vi "Spark MAX_Get ALL Cached Parameter.vi"(8 "error in (no error)":errorcluster, 10 "Parameter ID":T2, 11 "SPARK MAX Device Ref in":T4) -> (0 "error out":errorcluster, 1 "Parameter Type":T3, 2 "Parameter Raw":u32, 3 "output cluster":T1 {"Float" format="%#_4f"}, 5 "Timestamp":u32)   [LabVIEW 2020]
uses:
  <vilib>/Rock Robotics/WPI/ThirdParty/REV Robotics/REVLib/Typedef/Spark MAX Parameter Type.ctl
  <vilib>/Rock Robotics/WPI/ThirdParty/REV Robotics/REVLib/Typedef/Spark MAX Parameter ID.ctl
  <vilib>/Rock Robotics/WPI/ThirdParty/REV Robotics/REVLib/Typedef/Spark MAX Variant Data.ctl
  Cluster_Spark Max parameter data.ctl
  <vilib>/Rock Robotics/WPI/ThirdParty/REV Robotics/REVLib/Typedef/Spark MAX Parameter Cache Element.ctl
  <vilib>/Rock Robotics/WPI/ThirdParty/REV Robotics/REVLib/Typedef/Spark MAX Parameter Status.ctl
panel:
  out "found":bool
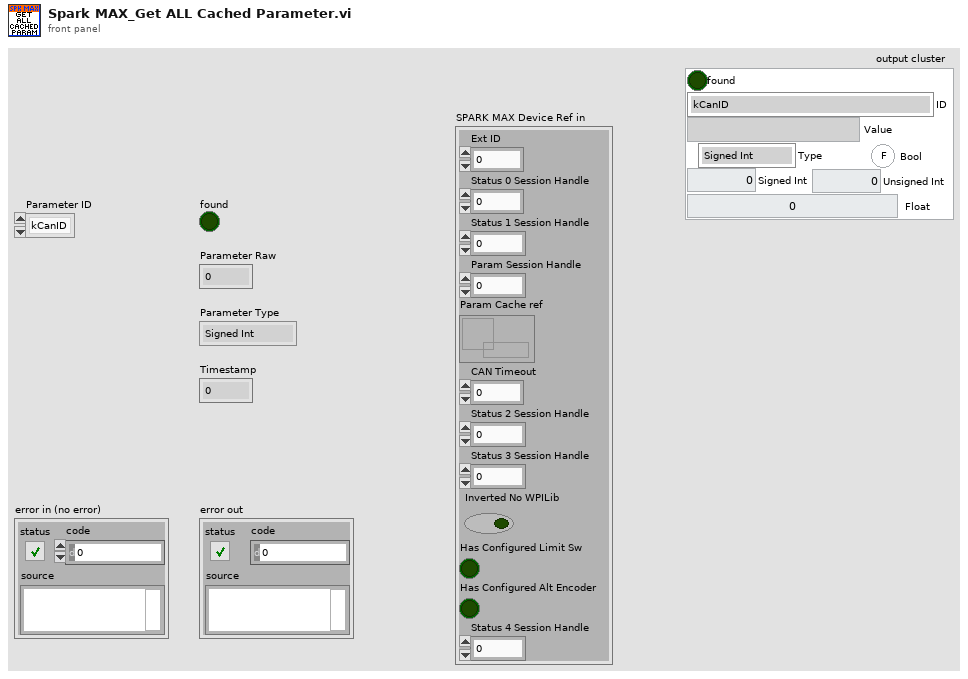
[diagram p1: front panel]
types:
  T1 = typedef "Cluster_Spark Max parameter data.ctl" = cluster{"found":bool, "ID":T2, "Value":string, "Type":T3, "Signed Int":i32, "Unsigned Int":u32, "Float":dbl, "Bool":bool}
  T2 = typedef "Spark MAX Parameter ID.ctl" = enum16{"kCanID", "kInputMode", "kMotorType", "kCommAdvance", "kSensorType", "kCtrlType", "kIdleMode", "kInputDeadband", "kFeedbackSensorPID0", "kFeedbackSensorPID1", "kPolePairs", "kCurrentChop", "kCurrentChopCycles", "kP_0", "kI_0", "kD_0", "kF_0", "kIZone_0", "kDFilter_0", "kOutputMin_0", "kOutputMax_0", "kP_1", "kI_1", "kD_1", "kF_1", "kIZone_1", "kDFilter_1", "kOutputMin_1", "kOutputMax_1", "kP_2", "kI_2", "kD_2", "kF_2", "kIZone_2", "kDFilter_2", "kOutputMin_2", "kOutputMax_2", "kP_3", "kI_3", "kD_3", "kF_3", "kIZone_3", "kDFilter_3", "kOutputMin_3", "kOutputMax_3", "kInverted", "kOutputRatio", "kSerialNumberLow", "kSerialNumberMid", "kSerialNumberHigh", "kLimitSwitchFwdPolarity", "kLimitSwitchRevPolarity", "kHardLimitFwdEn", "kHardLimitRevEn", "kSoftLimitFwdEn", "kSoftLimitRevEn", "kRampRate", "kFollowerID", "kFollowerConfig", "kSmartCurrentStallLimit", "kSmartCurrentFreeLimit", "kSmartCurrentConfig", "kSmartCurrentReserved", "kMotorKv", "kMotorR", "kMotorL", "kMotorRsvd1", "kMotorRsvd2", "kMotorRsvd3", "kEncoderCountsPerRev", "kEncoderAverageDepth", "kEncoderSampleDelta", "kEncoderInverted", "kEncoderRsvd1", "kClosedLoopVoltageMode", "kCompensatedNominalVoltage", "kSmartMotionMaxVelocity_0", "kSmartMotionMaxAccel_0", "kSmartMotionMinVelOutput_0", "kSmartMotionAllowedClosedLoopError_0", "kSmartMotionAccelStrategy_0", "kSmartMotionMaxVelocity_1", "kSmartMotionMaxAccel_1", "kSmartMotionMinVelOutput_1", "kSmartMotionAllowedClosedLoopError_1", "kSmartMotionAccelStrategy_1", "kSmartMotionMaxVelocity_2", "kSmartMotionMaxAccel_2", "kSmartMotionMinVelOutput_2", "kSmartMotionAllowedClosedLoopError_2", "kSmartMotionAccelStrategy_2", "kSmartMotionMaxVelocity_3", "kSmartMotionMaxAccel_3", "kSmartMotionMinVelOutput_3", "kSmartMotionAllowedClosedLoopError_3", "kSmartMotionAccelStrategy_3", "kIMaxAccum_0", "kSlot3Placeholder1_0", "kSlot3Placeholder2_0", "kSlot3Placeholder3_0", "kIMaxAccum_1", "kSlot3Placeholder1_1", "kSlot3Placeholder2_1", "kSlot3Placeholder3_1", "kIMaxAccum_2", "kSlot3Placeholder1_2", "kSlot3Placeholder2_2", "kSlot3Placeholder3_2", "kIMaxAccum_3", "kSlot3Placeholder1_3", "kSlot3Placeholder2_3", "kSlot3Placeholder3_3", "kPositionConversionFactor", "kVelocityConversionFactor", "kClosedLoopRampRate", "kSoftLimitFwd", "kSoftLimitRev", "kSoftLimitRsvd0", "kSoftLimitRsvd1", "kAnalogPositionConversion", "kAnalogVelocityConversion", "kAnalogAverageDepth", "kAnalogSensorMode", "kAnalogInverted", "kAnalogSampleDelta", "kAnalogRsvd0", "kAnalogRsvd1", "kDataPortConfig", "kAltEncoderCountsPerRev", "kAltEncoderAverageDepth", "kAltEncoderSampleDelta", "kAltEncoderInverted", "kAltEncoderPositionConversion", "kAltEncoderVelocityConversion", "kAltEncoderRsvd0", "kAltEncoderRsvd1", "kHallSensorSampleRate", "kHallSensorAverageDepth", "kNumParameters", "kDutyCyclePositionFactor", "kDutyCycleVelocityFactor", "kDutyCycleInverted", "kDutyCycleSensorMode", "kDutyCycleAverageDepth", "kDutyCycleSampleDelta", "kDutyCycleOffsetv1p6p2", "kDutyCycleRsvd0", "kDutyCycleRsvd1", "kDutyCycleRsvd2", "kPositionPIDWrapEnable", "kPositionPIDMinInput", "kPositionPIDMaxInput", "kDutyCycleZeroCentered", "kDutyCyclePrescalar", "kDutyCycleOffset"}
  T3 = typedef "Spark MAX Parameter Type.ctl" = enum16{"Signed Int", "Unsigned Int", "Float", "Bool"}
  T4 = typedef "Spark MAX Variant Data.ctl" = cluster{"Ext ID":u32, "Status 0 Session Handle":u32, "Status 1 Session Handle":u32, "Param Session Handle":u32, "Param Cache ref":refnum<data-value>, "CAN Timeout":u32, "Status 2 Session Handle":u32, "Status 3 Session Handle":u32, "Inverted No WPILib":bool, "Has Configured Limit Sw":bool, "Has Configured Alt Encoder":bool, "Status 4 Session Handle":u32}
  T5 = typedef "Spark MAX Parameter Status.ctl" = enum16{"Ok", "Invalid Parameter ID", "Mismatch Type", "Access Mode", "Invalid Parameter Value", "Not Implemented/Depcrecated"}
  T6 = typedef "Spark MAX Parameter Cache Element.ctl" = cluster{"Timestamp":u32, "Parameter Raw":u32, "Parameter Type":T3, "Last Access Status":T5}
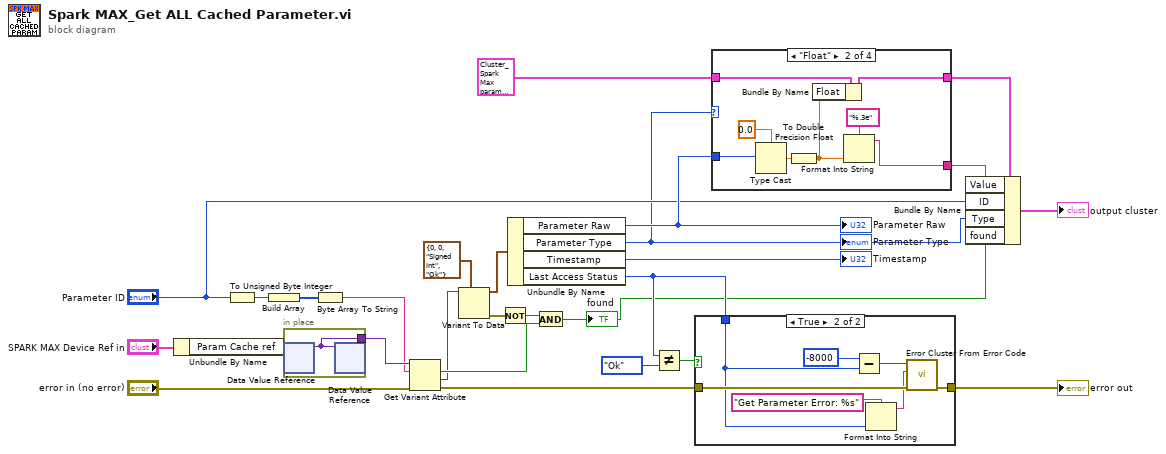
[diagram p0: block diagram]
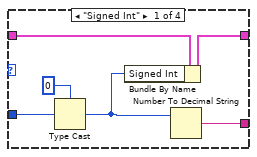
[diagram p2: hidden frame]
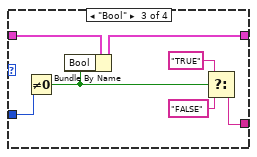
[diagram p3: hidden frame]
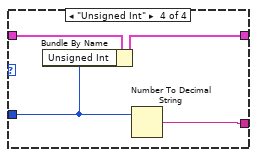
[diagram p4: hidden frame]
diagram:
  n1 = Unbundle By Name("SPARK MAX Device Ref in") -> ("Param Cache ref"=w15:refnum<data-value>)
  n2 = To Unsigned Byte Integer(number="Parameter ID") -> (unsigned 8bit integer=w19:u8)
  n3 = Build Array(w19) -> (w17:u8[])
  n4 = in-place {
    in-place-border: [w28] -> w14
    n5 = in-place-dvr #1(w15) -> (w28:variant)  [unwired: 1 out]
    n6 = in-place-dvr #1(w28) -> ()  [unwired: 2 out]
  }
  n7 = Byte Array To String(unsigned byte array=w17) -> (string=w13:string)
  n8 = Get Variant Attribute(Variant=w14, name=w13, error in="error in (no error)") -> (found=w23:bool, value=w21:variant, error out=w25:errorcluster)  [unwired: 1 in, 1 out]
  n9 = Variant To Data(type=T6 {"Timestamp"=0, "Parameter Raw"=0, "Parameter Type"=enum."Signed Int", "Last Access Status"=enum."Ok"} ("Cluster"), Variant=w21) -> (data=w26:T6, error out=w22:errorcluster)  [unwired: 1 in]
  n10 = Not(x=w22) -> (.not. x?=w24:bool)
  n11 = Unbundle By Name(w26) -> ("Parameter Raw"=w8:u32, "Parameter Type"=w4:T3, "Timestamp"=→"Timestamp":u32, "Last Access Status"=w11:T5)
  "Parameter Raw" <- w8
  "Parameter Type" <- w4
  n12 = And(x=w24, y=w23) -> (x .and. y?=w3:bool)
  "found" <- w3
  n13 = Not Equal?(x=w11, y=Spark_MAX_Parameter_Status."Ok") -> (x != y?=w10:bool)
  n14 = case shown="True" w10 {
    tunnel: w25 -> [w29 w36]
    tunnel: [w29 w35] -> w12
    tunnel: w11 -> [_ w32]
    frame False {
    }
    frame True {
      n15 = Subtract(x=-8000 ("error code (0)"), y=w32) -> (x-y=w33:i32)
      n16 = Format Into String(format string="Get Parameter Error: %s", w32) -> (resulting string=w31:string)  [unwired: 2 in, 1 out]
      n17 = call <vilib>:"Error Cluster From Error Code.vi"("error in (no error)"=w36, "error message (\"\")"=w31, "error code (0)"=w33) -> ("error out"=w35:errorcluster)  [unwired: 6 in]
    }
  }
  "error out" <- w12
  n18 = case shown="\"Float\"" w4 {
    tunnel: w8 -> [w42 w50 w57 w58]
    tunnel: [w40 w46 w54 w61] -> w6
    tunnel: T1 {"found"=FALSE, "ID"=enum."kSmartMotionAllowedClosedLoopError_0", "Value"="", "Type"=enum."Signed Int", "Signed Int"=0, "Unsigned Int"=0, "Float"=0.0, "Bool"=FALSE} ("Spark Max Parameter") -> [w39 w45 w53 w59]
    tunnel: [w38 w44 w52 w60] -> w1
    frame "Signed Int" {
      n19 = Type Cast(type=0, x=w42) -> (*(type *) &x=w37:i32)
      n20 = Bundle By Name(cluster=w39, "Signed Int"=w37) -> (w38:T1)
      n21 = Number To Decimal String(number=w37) -> (decimal integer string=w40:string)  [unwired: 1 in]
    }
    frame "Float" {
      n22 = Type Cast(type=sgl 0.0, x=w50) -> (*(type *) &x=w48:sgl)
      n23 = To Double Precision Float(number=w48) -> (double precision float=w43:dbl)
      n24 = Bundle By Name(cluster=w45, "Float"=w43) -> (w44:T1)
      n25 = Format Into String(format string="%.3e", w43) -> (resulting string=w46:string)  [unwired: 2 in, 1 out]
    }
    frame "Bool" {
      n26 = Not Equal To 0?(x=w57) -> (x != 0?=w51:bool)
      n27 = Bundle By Name(cluster=w53, "Bool"=w51) -> (w52:T1)
      n28 = Select(t="TRUE", s=w51, f="FALSE") -> (s? t:f=w54:string)
    }
    frame "Unsigned Int" {
      n29 = Bundle By Name(cluster=w59, "Unsigned Int"=w58) -> (w60:T1)
      n30 = Number To Decimal String(number=w58) -> (decimal integer string=w61:string)  [unwired: 1 in]
    }
  }
  n31 = Bundle By Name(cluster=w1, "Value"=w6, "ID"="Parameter ID", "Type"=w4, "found"=w3) -> (→"output cluster":T1)
